vi "Plot_Channels.vi"() -> (5 "Plug in titles":string[](array[string]), 7 "Plug in values":string[](array[string]))   [LabVIEW 2011]
uses:
  Globals/Meas_global.vi
panel:
  out "Size 2":i32
  out "Size 1":i32
  out "Size 0":i32
  in  "index 2":i32=3
  out "XY Graph":cluster{"Time (ms)":dbl[], "Eng Values":dbl[]}[](graph)
  in  "index 1":i32=1
  in  "index 0":i32
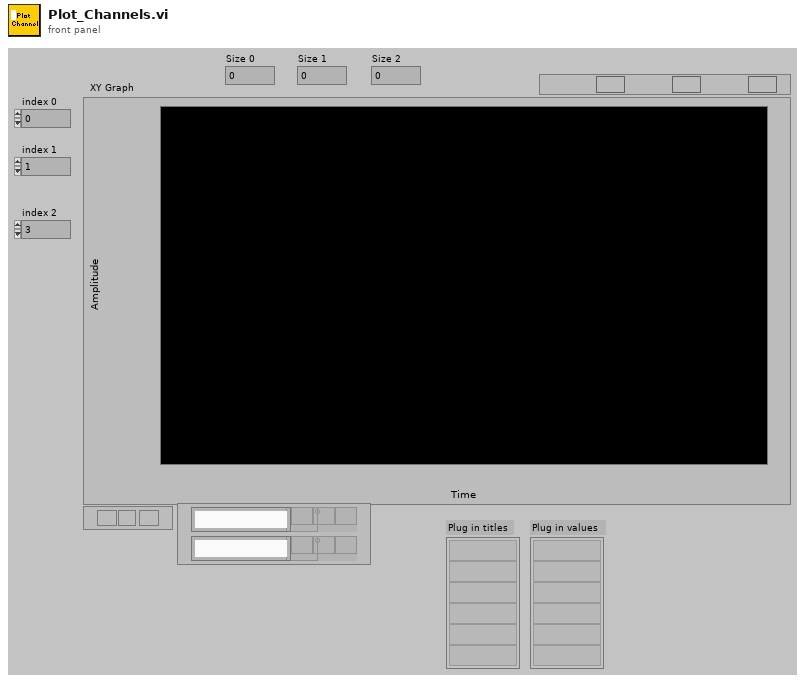
[diagram p1: front panel]
types:
  T1 = typedef "Analysis_info_cluster.ctl" = cluster{"Colour":u32, "Inst type":T2, "Inst name":string, "Symbol":string, "Code name":string, "Extra Info":string, "Inst Array":T3, "Index":i32, "Voltage Index":i32, "Extra Titles":string[], "Extra Values":string[], "Eng Values":dbl[], "Time (ms)":dbl[], "Voltage":dbl[], "U":dbl, "u^2":dbl, "u^3":dbl, "u^4":dbl, "Skew_u":dbl, "Kurt_u":dbl, "Sd Error in Mean":dbl, "% u'/U":dbl, "X":dbl, "Y":dbl, "Z":dbl, "Spectra":T4, "Autocorrelation":T4, "Timescale integral to 25%":dbl, "Sd Error in Variance":dbl, "Calib File":path, "Calib Constants":dbl[], "Histogram":T4, "Output Position":bool, "Full Stats":bool, "Weighting":dbl[]}
  T2 = typedef "Inst_type.ctl" = enum16{"Propeller anemometer", "Raw voltage", "Pressure Transducer", "Pitot-static tube", "Preston tube", "Hot wire", "Cross wire 1", "Cross wire 2", "Generic Linear", "Generic Polynomial", "Generic BackPoly", "Fast FID", "Thermocouple", "Cold wire", "Pulsed Wire", "LDA Vel", "LDA Tran time", "LDA Arr time"}
  T3 = typedef "Instrument_Array.ctl" = enum16{"PWA", "LDA", "Analogue"}
  T4 = typedef "XY_Plot_Cluster.ctl" = cluster{"First Name":string, "Second Name":string, "X axis name":string, "Y axis name":string, "X array":dbl[], "Y array":dbl[]}
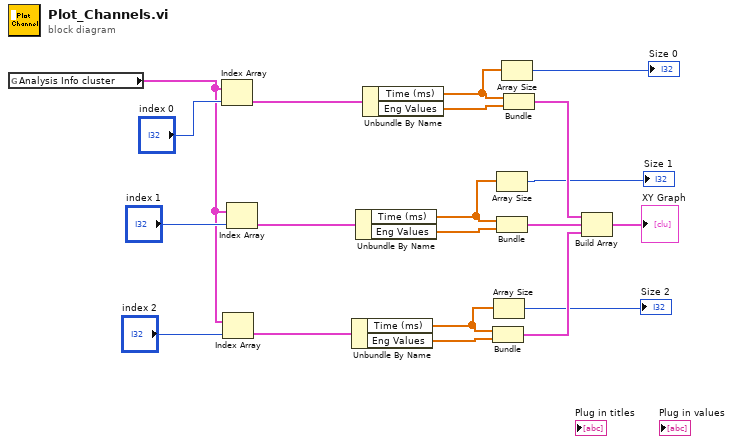
[diagram p0: block diagram]
diagram:
  n1 = global read "Meas_global.vi" "Analysis Info cluster"() -> (w4:T1[])
  n2 = Index Array(array=w4, index="index 0") -> (element=w1:T1)
  n3 = Index Array(array=w4, index="index 2") -> (element=w3:T1)
  n4 = Index Array(array=w4, index="index 1") -> (element=w2:T1)
  n5 = Unbundle By Name(w3) -> ("Time (ms)"=w8:dbl[], "Eng Values"=w13:dbl[])
  n6 = Unbundle By Name(w2) -> ("Time (ms)"=w9:dbl[], "Eng Values"=w17:dbl[])
  n7 = Unbundle By Name(w1) -> ("Time (ms)"=w10:dbl[], "Eng Values"=w18:dbl[])
  n8 = Bundle("Time (ms)"=w8, "Eng Values"=w13) -> (w11:cluster{"Time (ms)":dbl[], "Eng Values":dbl[]})  [unwired: 1 in]
  n9 = Array Size(array=w8) -> (size(s)=→"Size 2":i32)
  n10 = Array Size(array=w9) -> (size(s)=→"Size 1":i32)
  n11 = Bundle("Time (ms)"=w9, "Eng Values"=w17) -> (w16:cluster{"Time (ms)":dbl[], "Eng Values":dbl[]})  [unwired: 1 in]
  n12 = Array Size(array=w10) -> (size(s)=→"Size 0":i32)
  n13 = Bundle("Time (ms)"=w10, "Eng Values"=w18) -> (w15:cluster{"Time (ms)":dbl[], "Eng Values":dbl[]})  [unwired: 1 in]
  n14 = Build Array(w15, w16, w11) -> (→"XY Graph":cluster{"Time (ms)":dbl[], "Eng Values":dbl[]}[])
